vi "Returning Values By Reference Simple Struct.vi"(7 "largerCircle":cluster{"x":sgl, "y":sgl, "radius":sgl}, 8 "error in (no error)":errorcluster, 9 "radius":sgl, 10 "y":sgl, 11 "x":sgl) -> (0 "error out":errorcluster, 5 "largerCircle out":cluster{"x":sgl, "y":sgl, "radius":sgl})   [LabVIEW 2009, in "LabVIEWWrapper_PassingDataSampleDLL.lvlib"]
doc: "void ReturningValuesByReference_SimpleStruct (struct simpleStructCircle circle, struct simpleStructCircle *largerCircle);"
uses:
  LabVIEWWrapper_PassingDataSampleDLL.lvlib
  PassingDataSampleDLL.dll
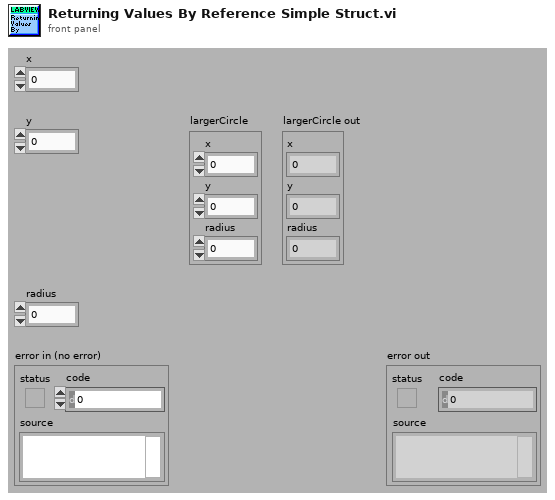
[diagram p1: front panel]
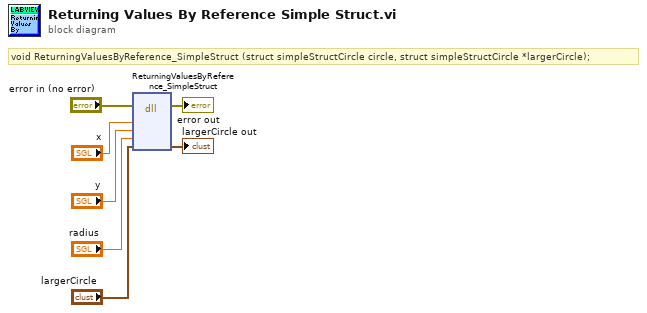
[diagram p0: block diagram]
diagram:
  # "void ReturningValuesByReference_SimpleStruct (struct simpleStructCircle circle, struct simpleStructCircle *largerCircle);"
  n1 = dll-call lib="C:/My Dropbox/Systems Engineering Application/SDK/C Integration/LabVIEWWrapper/PassingDataSampleDLL.*" fn="ReturningValuesByReference_SimpleStruct"(error in="error in (no error)", "x"="x", "y"="y", "radius"="radius", "largerCircle"="largerCircle") -> (error out=→"error out":errorcluster, "largerCircle"=→"largerCircle out":cluster{"x":sgl, "y":sgl, "radius":sgl})  [unwired: 6 in, 1 out]
